vi "Get All Attributes.vi"(8 "error in":errorcluster, 10 "Section Node":refnum<k20>, 11 "Section Ref in":refnum<data-value>) -> (0 "error out":errorcluster, 3 "Section Ref out":refnum<data-value>)   [LabVIEW 2024, in "Config File Parser.lvlib" / "Section.lvclass"]
uses:
  Section.lvclass
  Section.lvclass/Section.ctl
  <vilib>/xml/Close Reference(Node).vi
  <resource>/objmgr/DOMUserDefRef.rc
  <vilib>/xml/NI_XML.lvlib
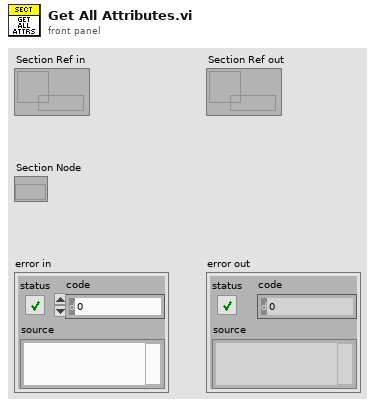
[diagram p1: front panel]
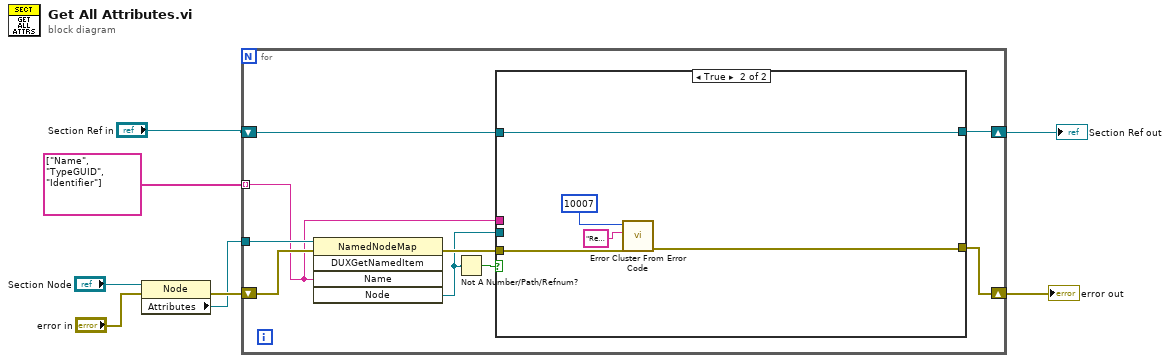
[diagram p0: block diagram]
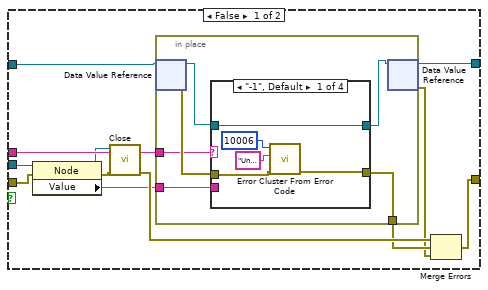
[diagram p2: hidden frame]
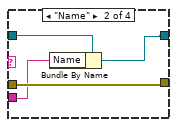
[diagram p3: hidden frame]
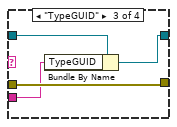
[diagram p4: hidden frame]
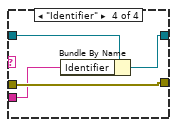
[diagram p5: hidden frame]
diagram:
  n1 = property class="Node"(reference="Section Node", error in="error in") -> (error out=w7:errorcluster, "Attributes"=w4:refnum<k20>)  [unwired: 1 out]
  n2 = for {
    tunnel: w4 -> [w14]
    shift-right: [w15] -> w6
    shift-left: w7 -> [w17]
    tunnel: string[] ["Name", "TypeGUID", "Identifier"] -> [w13] mode=indexing
    shift-right: [w10] -> w1
    shift-left: "Section Ref in" -> [w9]
    n3 = invoke class="NamedNodeMap" method="DUXGetNamedItem"(reference=w14, error in=w17, "Name"=w13) -> (error out=w16:errorcluster, "Node"=w11:refnum<k20>)  [unwired: 2 in, 3 out]
    n4 = Not A Number/Path/Refnum?(number/path/refnum=w11) -> (NaN/Path/Refnum?=w12:bool)
    n5 = case shown="True" w12 {
      tunnel: w13 -> [w23 _]
      tunnel: w11 -> [w22 _]
      tunnel: w16 -> [w28 w57]
      tunnel: [w24 w56] -> w15
      tunnel: [w19 w53] -> w10
      tunnel: w9 -> [w18 w53]
      frame False {
        n6 = property class="Node"(reference=w22, error in=w28) -> (reference out=w20:refnum<k20>, error out=w29:errorcluster, "Value"=w21:string)
        n7 = call-poly <vilib>:"Close.vi"("error in (no error)"=w29, "node"=w20) -> ("error out"=w27:errorcluster)  [unwired: 7 in]
        n8 = in-place {
          in-place-border: w23 -> [w33]
          in-place-border: w21 -> [w32]
          in-place-border: [w34] -> w26
          n9 = in-place-dvr #1(w18) -> (w31:refnum<class "Section.lvclass">, w35:errorcluster)
          n10 = case shown="\"-1\", Default" w33 {
            tunnel: w31 -> [w37 w42 w46 w50]
            tunnel: [w37 w41 w45 w49] -> w30
            tunnel: w32 -> [_ w43 w47 w51]
            tunnel: w35 -> [w40 w44 w48 w52]
            tunnel: [w39 w44 w48 w52] -> w34
            frame "-1", Default {
              n11 = call <vilib>:"Error Cluster From Error Code.vi"("error in (no error)"=w40, "error message (\"\")"="Unauthorized attributes are found. The section should not contain any unauthorized attributes.", "error code (0)"=10006) -> ("error out"=w39:errorcluster)  [unwired: 6 in]
            }
            frame "Name" {
              n12 = Bundle By Name(cluster=w42, "Name"=w43) -> (w41:refnum<class "Section.lvclass">)
            }
            frame "TypeGUID" {
              n13 = Bundle By Name(cluster=w46, "TypeGUID"=w47) -> (w45:refnum<class "Section.lvclass">)
            }
            frame "Identifier" {
              n14 = Bundle By Name(cluster=w50, "Identifier"=w51) -> (w49:refnum<class "Section.lvclass">)
            }
          }
          n15 = in-place-dvr #1(w30) -> (w19:refnum<data-value>, w25:errorcluster)
        }
        n16 = Merge Errors(w27, w26, w25) -> (w24:errorcluster)
      }
      frame True {
        n17 = call <vilib>:"Error Cluster From Error Code.vi"("error in (no error)"=w57, "error message (\"\")"="Required attributes are missing from the section", "error code (0)"=10007) -> ("error out"=w56:errorcluster)  [unwired: 6 in]
      }
    }
  }
  "error out" <- w6
  "Section Ref out" <- w1
